vi "Logging.vi"(0 "Main Image":T2, 1 "Particle Analysis":T2, 3 "Index":dbl, 4 "sorted array 2":T1(array[cluster])=[{"Particle Report"={"Area"=8785.0, "Number of Holes"=0.0, "Bounding Rect"={"Left"=787.0, "Top"=236.0, "Right"=913.0, "Bottom"=327.0}, "Center of Mass"={"X"=847.3036994877632, "Y"=282.0883323847467}, "Orientation"=2.357887159702958, "Dimensions"={"Width"=126.0, "Height"=91.0}}, "angle"=-101.58703756402963, "Distance"=2.2387148939763}, {"Particle Report"={"Area"=4202.0, "Number of Holes"=0.0, "Bounding Rect"={"Left"=1224.0, "Top"=126.0, "Right"=1316.0, "Bottom"=196.0}, "Center of Mass"={"X"=1268.6087577344122, "Y"=161.86625416468348}, "Orientation"=29.688425464358808, "Dimensions"={"Width"=92.0, "Height"=70.0}}, "angle"=-48.92390528319845, "Distance"=5.080592942706545}, {"Particle Report"={"Area"=3897.0, "Number of Holes"=0.0, "Bounding Rect"={"Left"=1406.0, "Top"=109.0, "Right"=1490.0, "Bottom"=193.0}, "Center of Mass"={"X"=1447.0959712599436, "Y"=153.37002822684116}, "Orientation"=48.522436035724326, "Dimensions"={"Width"=84.0, "Height"=84.0}}, "angle"=-26.613003592507084, "Distance"=5.481555651547687}, {"Particle Report"={"Area"=2595.0, "Number of Holes"=0.0, "Bounding Rect"={"Left"=1818.0, "Top"=102.0, "Right"=1882.0, "Bottom"=161.0}, "Center of Mass"={"X"=1848.9445086705202, "Y"=132.05472061657034}, "Orientation"=40.73277035999637, "Dimensions"={"Width"=64.0, "Height"=59.0}}, "angle"=23.61806358381503, "Distance"=6.759742610507792}, {"Particle Report"={"Area"=2210.0, "Number of Holes"=0.0, "Bounding Rect"={"Left"=1564.0, "Top"=130.0, "Right"=1623.0, "Bottom"=178.0}, "Center of Mass"={"X"=1591.7723981900454, "Y"=154.22262443438913}, "Orientation"=8.230110141050458, "Dimensions"={"Width"=59.0, "Height"=48.0}}, "angle"=-8.528450226244331, "Distance"=5.438986022082759}, {"Particle Report"={"Area"=2156.0, "Number of Holes"=0.0, "Bounding Rect"={"Left"=1328.0, "Top"=93.0, "Right"=1403.0, "Bottom"=143.0}, "Center of Mass"={"X"=1365.550556586271, "Y"=118.6734693877551}, "Orientation"=156.04787613526668, "Dimensions"={"Width"=75.0, "Height"=50.0}}, "angle"=-36.80618042671614, "Distance"=7.847284436452411}, {"Particle Report"={"Area"=1561.0, "Number of Holes"=0.0, "Bounding Rect"={"Left"=1903.0, "Top"=110.0, "Right"=1951.0, "Bottom"=150.0}, "Center of Mass"={"X"=1926.144138372838, "Y"=130.42216527866753}, "Orientation"=1.0600188419131478, "Dimensions"={"Width"=48.0, "Height"=40.0}}, "angle"=33.26801729660474, "Distance"=6.878227161223234}, {"Particle Report"={"Area"=1046.0, "Number of Holes"=0.0, "Bounding Rect"={"Left"=1026.0, "Top"=103.0, "Right"=1068.0, "Bottom"=135.0}, "Center of Mass"={"X"=1045.9273422562142, "Y"=119.6434034416826}, "Orientation"=179.6787354639328, "Dimensions"={"Width"=42.0, "Height"=32.0}}, "angle"=-76.75908221797323, "Distance"=7.758593842607151}, {"Particle Report"={"Area"=1040.0, "Number of Holes"=0.0, "Bounding Rect"={"Left"=1616.0, "Top"=97.0, "Right"=1657.0, "Bottom"=130.0}, "Center of Mass"={"X"=1635.3480769230769, "Y"=113.49230769230769}, "Orientation"=8.78851402048618, "Dimensions"={"Width"=41.0, "Height"=33.0}}, "angle"=-3.0814903846153925, "Distance"=8.352241095610436}], 5 "refnum out":refnum<file>, 7 "Path":path) -> ()   [LabVIEW 2025]
uses:
  <vilib>/vision/Image Controls.llb/IMAQ Image.ctl
panel:
  out "error out":errorcluster
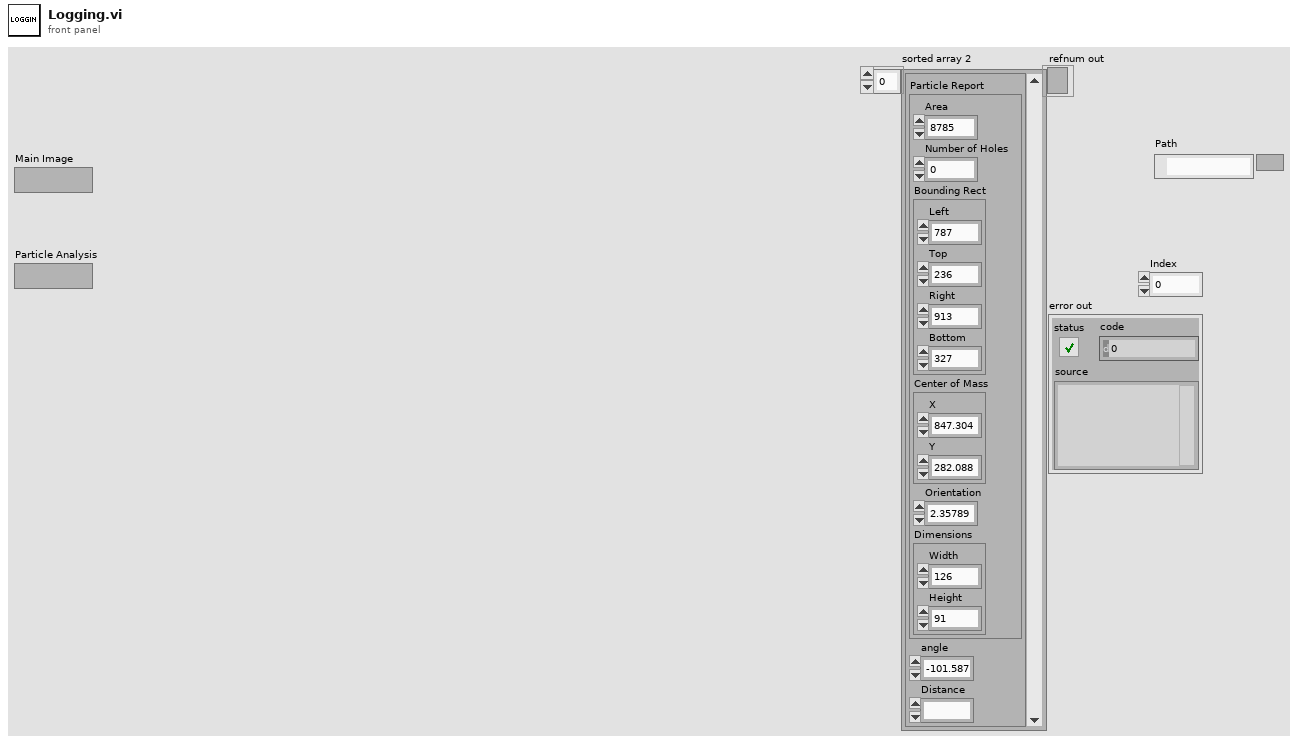
[diagram p1: front panel]
types:
  T1 = cluster{"Particle Report":cluster{"Area":dbl, "Number of Holes":dbl, "Bounding Rect":cluster{"Left":dbl, "Top":dbl, "Right":dbl, "Bottom":dbl}, "Center of Mass":cluster{"X":dbl, "Y":dbl}, "Orientation":dbl, "Dimensions":cluster{"Width":dbl, "Height":dbl}}, "angle":dbl, "Distance":ext}[]
  T2 = typedef "IMAQ Image.ctl" = refnum<image>
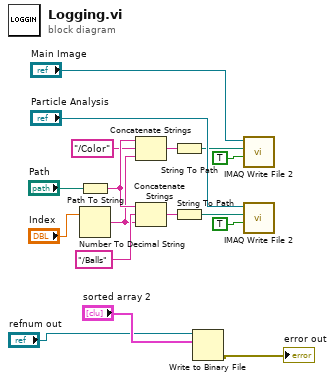
[diagram p0: block diagram]
diagram:
  n1 = Path To String(path="Path") -> (string=w9:string)
  n2 = Number To Decimal String(number="Index") -> (decimal integer string=w6:string)  [unwired: 1 in]
  n3 = Concatenate Strings(w9, "/Color" ("string"), w6) -> (w5:string)
  n4 = Concatenate Strings(w9, "/Balls" ("string"), w6) -> (w3:string)
  n5 = String To Path(string=w5) -> (path=w4:path)
  n6 = String To Path(string=w3) -> (path=w2:path)
  n7 = Write to Binary File(file (use dialog)="refnum out", data="sorted array 2") -> (error out=→"error out":errorcluster)  [unwired: 4 in, 2 out]
  n8 = call-poly "IMAQ Write File 2"("Compress? (N)"=TRUE, "File Path"=w4, "Image"="Main Image") -> ()  [unwired: 7 in, 2 out]
  n9 = call-poly "IMAQ Write File 2"("Compress? (N)"=TRUE, "File Path"=w2, "Image"="Particle Analysis") -> ()  [unwired: 7 in, 2 out]
